vi "Process Transmission Request.vi"(8 "error in (no error)":errorcluster, 10 "Write Request":T1, 11 "Network Session Handler in":refnum<class "Network Session Handler.lvclass">) -> (0 "error out":errorcluster, 3 "Network Session Handler out":refnum<class "Network Session Handler.lvclass">)   [LabVIEW 2017, in "Network Interface.lvlib" / "Network Session Handler.lvclass"]
uses:
  <vilib>/gpm_packages/@cs/Network-sink/Source/Network Interface/Network Session Handler/Network Session Handler.lvclass
  <vilib>/gpm_packages/@cs/Network-sink/Source/Network Interface/Connection Handler/Synchronous Write Request.ctl
  <vilib>/gpm_packages/@cs/Network-sink/Source/Network Interface/Connection Handler/Message Names ENUM.ctl
  <vilib>/gpm_packages/@cs/event-logger/Source/Composed Log/Types/Log Level.ctl
  <vilib>/gpm_packages/@cs/Network-sink/Source/Network Interface/Network Session Handler/Network Session Handler.lvclass/Network Session Handler.ctl
  <vilib>/gpm_packages/@cs/event-logger/Source/Composed Log/LoggerReference/LoggerReference.lvclass/LoggerReference.ctl
  <vilib>/gpm_packages/@cs/event-logger/Source/Composed Log/LoggerReference/Log.vi
  <vilib>/gpm_packages/@cs/event-logger/Source/Composed Log/LoggerReference/Get Valid Event Time.vi
  <vilib>/gpm_packages/@cs/event-logger/Source/Composed Log/LoggerReference/Remove Stale Logs.vi
  <vilib>/Utility/error.llb/Error Cluster From Error Code.vi
  <vilib>/ErrorRing/Error Ring.xnode
  <vilib>/gpm_packages/@cs/Network-sink/Source/Network Interface/Connection Handler/Connection Handler.lvclass
  <vilib>/gpm_packages/@cs/event-logger/Source/Composed Log/Composed Log.lvlib
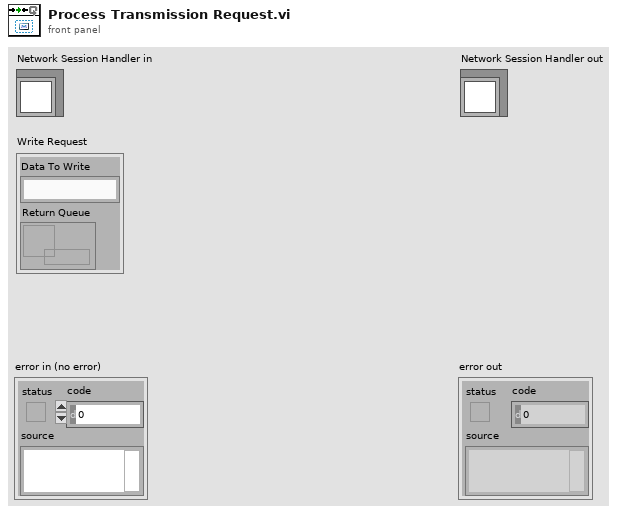
[diagram p1: front panel]
types:
  T1 = typedef "Network Interface.lvlib/Connection Handler.lvclass/Synchronous Write Request.ctl" = cluster{"Data To Write":string, "Return Queue":refnum<queue>}
  T2 = typedef "Composed Log.lvlib/Log Level.ctl" = enum16{"Debug", "Info", "Warning", "Error", "Critical"}
  T3 = typedef "Network Interface.lvlib/Connection Handler.lvclass/Message Names ENUM.ctl" = enum16{"Transmit Message", "Stop"}
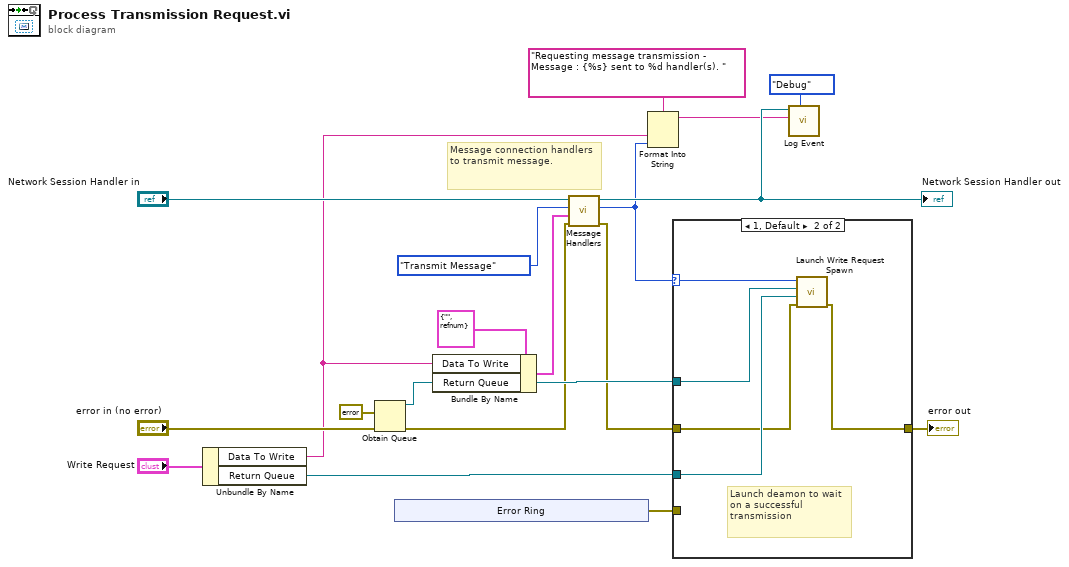
[diagram p0: block diagram]
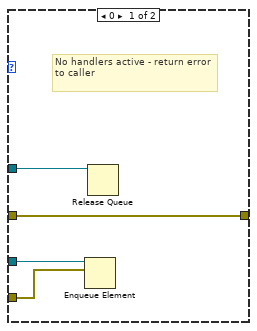
[diagram p2: hidden frame]
diagram:
  # "Message connection handlers to transmit message."
  n1 = Unbundle By Name("Write Request") -> ("Data To Write"=w2:string, "Return Queue"=w15:refnum<queue>)
  n2 = Obtain Queue(element data type=errorcluster {"status"=FALSE, "code"=0, "source"=""} ("error in (no error)"), error in (no error)="error in (no error)") -> (queue out=w16:refnum<queue>, error out=w8:errorcluster)  [unwired: 3 in, 1 out]
  n3 = xnode "Error Ring"() -> ("error out"=w12:errorcluster)
  n4 = Bundle By Name(cluster=T1 {"Data To Write"="", "Return Queue"=refnum} ("Write Request"), "Data To Write"=w2, "Return Queue"=w16) -> (w9:T1)
  n5 = call <vilib>:"Message Handlers.vi"("error in (no error)"=w8, "Message Data"=w9, "Message"=Message_Names_ENUM."Transmit Message", "Network Session Handler in"="Network Session Handler in") -> ("error out"=w7:errorcluster, "Number of Active Handlers"=w3:i32, "Network Session Handler out"=w6:refnum<class "Network Session Handler.lvclass">)  [unwired: 5 in]
  "Network Session Handler out" <- w6
  n6 = Format Into String(format string="Requesting message transmission - Message : {%s} sent to %d handler(s). ", w2, w3) -> (resulting string=w1:string)  [unwired: 2 in, 1 out]
  n7 = case shown="1, Default" w3 {
    selector: w3 -> [_ w28]
    tunnel: w16 -> [w22 w27]
    tunnel: w15 -> [w21 w26]
    tunnel: w7 -> [w23 w25]
    tunnel: [w23 w24] -> w13
    tunnel: w12 -> [w20 _]
    frame 0 {
      # "No handlers active - return error to caller"
      n8 = Enqueue Element(queue=w21, element=w20) -> ()  [unwired: 2 in, 3 out]
      n9 = Release Queue(queue=w22) -> ()  [unwired: 2 in, 3 out]
    }
    frame 1, Default {
      # "Launch deamon to wait on a successful transmission"
      n10 = call <vilib>:"Launch Write Request Spawn.vi"("error in (no error)"=w25, "Caller Return Queue"=w26, "Request Queue"=w27, "Number of Requests"=w28) -> ("error out"=w24:errorcluster)  [unwired: 7 in]
    }
  }
  "error out" <- w13
  n11 = call <vilib>:"Log Event.vi"("Event Level"=Log_Level."Debug", "Event"=w1, "Network Session Handler in"=w6) -> ()  [unwired: 7 in, 2 out]
